vi "RSZVB Save Color Scheme.vi"(8 "error in (no error)":errorcluster {"code" format="%.0x"}, 10 "File Name":string, 11 "VISA session":refnum<visa-resource-name>) -> (0 "error out":errorcluster {"code" format="%.0x"}, 3 "dup VISA session":refnum<visa-resource-name>)   [LabVIEW 2011]
doc: "This VI stores a color scheme to a specified NWA color scheme file.\n\nRemote-control command(s):\nMMEMory:STORe:CMAP '<file_name>'"
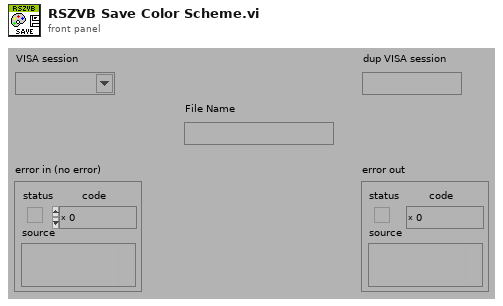
[diagram p1: front panel]
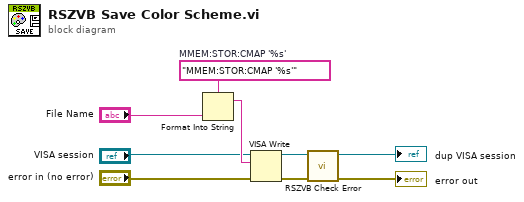
[diagram p0: block diagram]
diagram:
  w9 = "MMEM:STOR:CMAP '%s'"  # MMEM:STOR:CMAP '%s'
  n1 = Format Into String(format string=w9, "File Name") -> (resulting string=w6:string)  [unwired: 2 in, 1 out]
  n2 = VISA Write(VISA resource name="VISA session", write buffer=w6, error in (no error)="error in (no error)") -> (VISA resource name out=w7:refnum<visa-resource-name>, error out=w8:errorcluster)  [unwired: 1 out]
  n3 = call "RSZVB Check Error.vi"("error in (no error)"=w8, "VISA session"=w7) -> ("error out"=→"error out":errorcluster, "dup VISA session"=→"dup VISA session":refnum<visa-resource-name>)  [unwired: 8 in]
